vi "addressfinder.vi"() -> (3 "Subnet Local Broadcast Address":string)   [LabVIEW 2017]
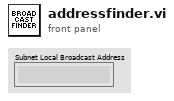
[diagram p1: front panel]
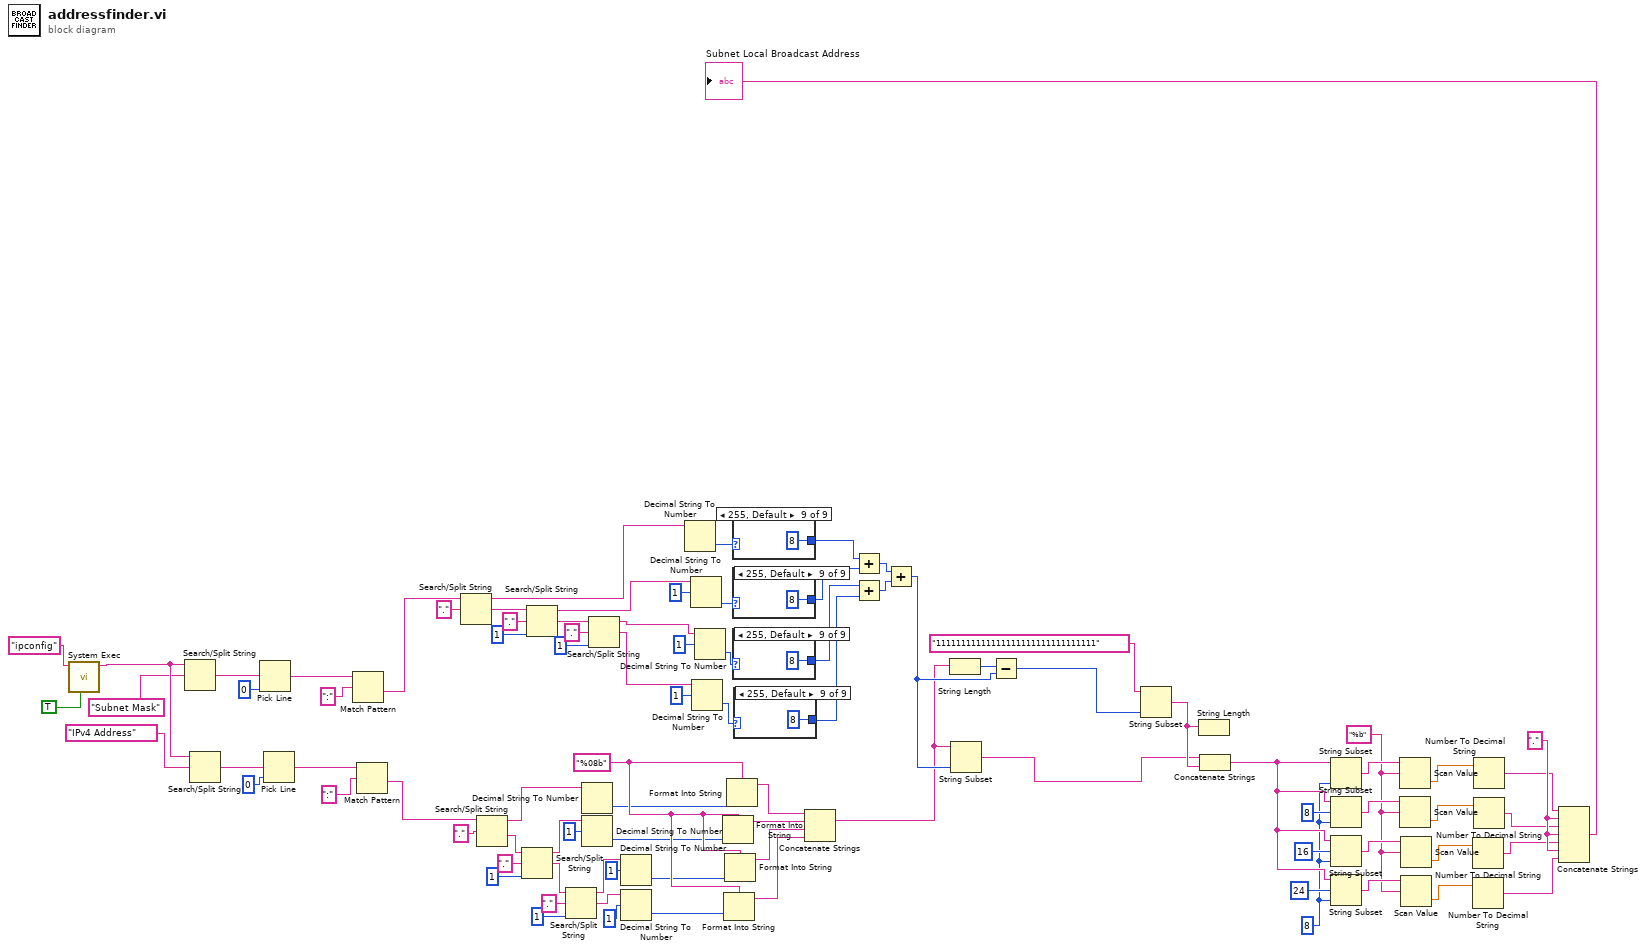
[diagram p0: block diagram]
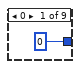
[diagram p2: hidden frame]
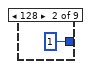
[diagram p3: hidden frame]
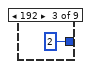
[diagram p4: hidden frame]
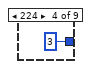
[diagram p5: hidden frame]
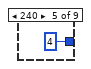
[diagram p6: hidden frame]
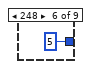
[diagram p7: hidden frame]
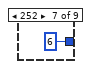
[diagram p8: hidden frame]
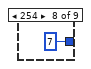
[diagram p9: hidden frame]
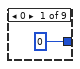
[diagram p10: hidden frame]
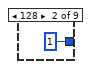
[diagram p11: hidden frame]
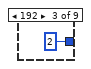
[diagram p12: hidden frame]
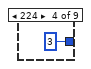
[diagram p13: hidden frame]
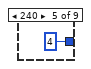
[diagram p14: hidden frame]
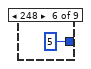
[diagram p15: hidden frame]
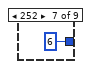
[diagram p16: hidden frame]
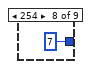
[diagram p17: hidden frame]
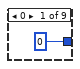
[diagram p18: hidden frame]
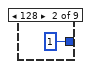
[diagram p19: hidden frame]
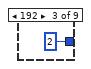
[diagram p20: hidden frame]
diagram:
  w88 = "."
  w75 = "%b" ("format string")
  w66 = 8
  w55 = "%08b" ("format string")
  n1 = call <vilib>:"System Exec.vi"("run minimized? (F)"=TRUE, "command line"="ipconfig") -> ("standard output"=w4:string)  [unwired: 6 in, 3 out]
  n2 = Search/Split String(string=w4, search string/char (-)="Subnet Mask") -> (match + rest of string=w6:string)  [unwired: 1 in, 2 out]
  n3 = Search/Split String(string=w4, search string/char (-)="IPv4 Address") -> (match + rest of string=w8:string)  [unwired: 1 in, 2 out]
  n4 = Pick Line(multi-line string=w6, line index=0) -> (output string=w10:string)  [unwired: 1 in]
  n5 = Pick Line(multi-line string=w8, line index=0) -> (output string=w12:string)  [unwired: 1 in]
  n6 = Match Pattern(string=w10, regular expression=":") -> (after substring=w14:string)  [unwired: 1 in, 3 out]
  n7 = Match Pattern(string=w12, regular expression=":") -> (after substring=w46:string)  [unwired: 1 in, 3 out]
  n8 = Search/Split String(string=w14, search string/char (-)=".") -> (substring before match=w22:string, match + rest of string=w17:string)  [unwired: 1 in, 1 out]
  n9 = Search/Split String(string=w46, search string/char (-)=".") -> (substring before match=w47:string, match + rest of string=w41:string)  [unwired: 1 in, 1 out]
  n10 = Search/Split String(string=w41, search string/char (-)=".", offset (0)=1) -> (substring before match=w52:string, match + rest of string=w45:string)  [unwired: 1 out]
  n11 = Search/Split String(string=w17, search string/char (-)=".", offset (0)=1) -> (substring before match=w23:string, match + rest of string=w21:string)  [unwired: 1 out]
  n12 = Search/Split String(string=w45, search string/char (-)=".", offset (0)=1) -> (substring before match=w53:string, match + rest of string=w54:string)  [unwired: 1 out]
  n13 = Decimal String To Number(string=w47) -> (number=w48:i32)  [unwired: 2 in, 1 out]
  n14 = Decimal String To Number(string=w52, offset=1) -> (number=w49:i32)  [unwired: 1 in, 1 out]
  n15 = Search/Split String(string=w21, search string/char (-)=".", offset (0)=1) -> (substring before match=w27:string, match + rest of string=w28:string)  [unwired: 1 out]
  n16 = Decimal String To Number(string=w53, offset=1) -> (number=w50:i32)  [unwired: 1 in, 1 out]
  n17 = Decimal String To Number(string=w54, offset=1) -> (number=w51:i32)  [unwired: 1 in, 1 out]
  n18 = Decimal String To Number(string=w22) -> (number=w29:i32)  [unwired: 2 in, 1 out]
  n19 = Decimal String To Number(string=w23, offset=1) -> (number=w30:i32)  [unwired: 1 in, 1 out]
  n20 = Decimal String To Number(string=w28, offset=1) -> (number=w32:i32)  [unwired: 1 in, 1 out]
  n21 = Decimal String To Number(string=w27, offset=1) -> (number=w31:i32)  [unwired: 1 in, 1 out]
  n22 = Format Into String(format string=w55, w49) -> (resulting string=w72:string)  [unwired: 2 in, 1 out]
  n23 = Format Into String(format string=w55, w51) -> (resulting string=w74:string)  [unwired: 2 in, 1 out]
  n24 = Format Into String(format string=w55, w50) -> (resulting string=w73:string)  [unwired: 2 in, 1 out]
  n25 = Format Into String(format string=w55, w48) -> (resulting string=w71:string)  [unwired: 2 in, 1 out]
  n26 = case shown="255, Default" w29 {
    tunnel: [0 1 2 3 4 5 6 7 8] -> w35
    frame 0 {
    }
    frame 128 {
    }
    frame 192 {
    }
    frame 224 {
    }
    frame 240 {
    }
    frame 248 {
    }
    frame 252 {
    }
    frame 254 {
    }
    frame 255, Default {
    }
  }
  n27 = case shown="255, Default" w30 {
    tunnel: [0 1 2 3 4 5 6 7 8] -> w36
    frame 0 {
    }
    frame 128 {
    }
    frame 192 {
    }
    frame 224 {
    }
    frame 240 {
    }
    frame 248 {
    }
    frame 252 {
    }
    frame 254 {
    }
    frame 255, Default {
    }
  }
  n28 = case shown="255, Default" w31 {
    tunnel: [0 1 2 3 4 5 6 7 8] -> w37
    frame 0 {
    }
    frame 128 {
    }
    frame 192 {
    }
    frame 224 {
    }
    frame 240 {
    }
    frame 248 {
    }
    frame 252 {
    }
    frame 254 {
    }
    frame 255, Default {
    }
  }
  n29 = case shown="255, Default" w32 {
    tunnel: [0 1 2 3 4 5 6 7 8] -> w38
    frame 0 {
    }
    frame 128 {
    }
    frame 192 {
    }
    frame 224 {
    }
    frame 240 {
    }
    frame 248 {
    }
    frame 252 {
    }
    frame 254 {
    }
    frame 255, Default {
    }
  }
  n30 = Concatenate Strings(w71, w72, w73, w74) -> (w59:string)
  n31 = Add(x=w35, y=w36) -> (x+y=w33:i32)
  n32 = Add(x=w37, y=w38) -> (x+y=w34:i32)
  n33 = Add(x=w33, y=w34) -> (x+y=w61:i32)
  n34 = String Length(string=w59) -> (length=w60:i32)
  n35 = String Subset(string=w59, length (rest)=w61) -> (substring=w64:string)  [unwired: 1 in]
  n36 = Subtract(x=w60, y=w61) -> (x-y=w62:i32)
  n37 = String Subset(string="11111111111111111111111111111111", length (rest)=w62) -> (substring=w65:string)  [unwired: 1 in]
  n38 = String Length(string=w65) -> ()  [unwired: 1 out]
  n39 = Concatenate Strings(w64, w65) -> (w70:string)
  n40 = String Subset(string=w70, length (rest)=w66) -> (substring=w76:string)  [unwired: 1 in]
  n41 = String Subset(string=w70, offset (0)=8, length (rest)=w66) -> (substring=w77:string)
  n42 = String Subset(string=w70, offset (0)=16, length (rest)=w66) -> (substring=w78:string)
  n43 = String Subset(string=w70, offset (0)=24, length (rest)=w66) -> (substring=w79:string)
  n44 = Scan Value(string=w76, format string=w75) -> (value=w80:dbl)  [unwired: 1 in, 1 out]
  n45 = Scan Value(string=w77, format string=w75) -> (value=w81:dbl)  [unwired: 1 in, 1 out]
  n46 = Scan Value(string=w78, format string=w75) -> (value=w82:dbl)  [unwired: 1 in, 1 out]
  n47 = Scan Value(string=w79, format string=w75) -> (value=w83:dbl)  [unwired: 1 in, 1 out]
  n48 = Number To Decimal String(number=w82) -> (decimal integer string=w86:string)  [unwired: 1 in]
  n49 = Number To Decimal String(number=w83) -> (decimal integer string=w87:string)  [unwired: 1 in]
  n50 = Number To Decimal String(number=w80) -> (decimal integer string=w84:string)  [unwired: 1 in]
  n51 = Number To Decimal String(number=w81) -> (decimal integer string=w85:string)  [unwired: 1 in]
  n52 = Concatenate Strings(w84, w88, w85, w88, w86, w88, w87) -> (→"Subnet Local Broadcast Address":string)
